vi "CmdSet_Async_OMAN.vi"(7 "nodeID":string, 10 "msg in":string) -> (2 "msg out":string)   [LabVIEW 2016]
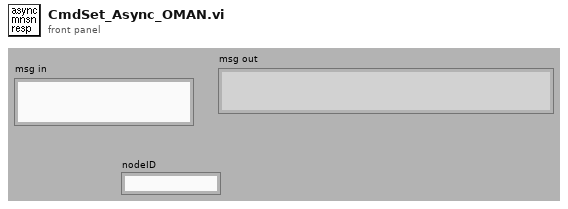
[diagram p1: front panel]
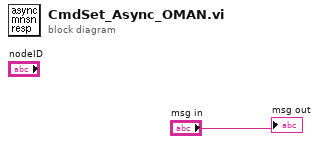
[diagram p0: block diagram]
diagram:
  "msg out" <- "msg in"
